vi "16TVTI-ReadITCStatus.vi"(0 "ITC IO Info":T1={"Com Port"=1, "ISOBUS Address"=1, "GPIB Address"=1, "Communication"=enum."ISOBUS"}) -> (2 "Control Channel":i16, 3 "System Status":i16, 4 "Auto heat":bool, 5 "ITC IO Info":T1={"Com Port"=1, "ISOBUS Address"=1, "GPIB Address"=1, "Communication"=enum."ISOBUS"}, 6 "Auto Needle Valve":bool, 8 "Sweeping":bool, 10 "Initialising Needle Valve":bool, 11 "Tuning?":bool, 13 "Auto PID":bool, 14 "Lock":bool, 15 "Remote":bool)   [LabVIEW 2019]
doc: "Reads the status of the ITC."
uses:
  Equipment/Oxford Software/Oxsoft/ITCSUBS.LLB/ITCIO.ctl
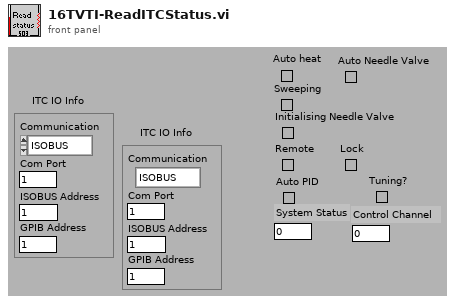
[diagram p1: front panel]
types:
  T1 = typedef "ITCIO.ctl" = cluster{"Com Port":i32, "ISOBUS Address":i32, "GPIB Address":i16, "Communication":enum16{"RS232", "ISOBUS", "GPIB", "Gateway"}}
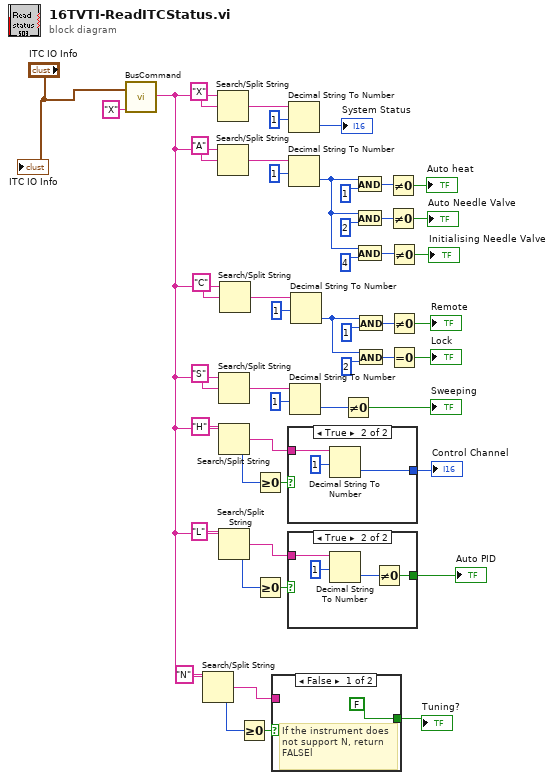
[diagram p0: block diagram]
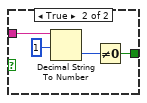
[diagram p2: hidden frame]
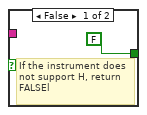
[diagram p3: hidden frame]
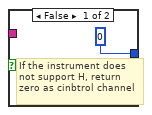
[diagram p4: hidden frame]
diagram:
  n1 = call "BusCommand.vi"("Command"="X", "Instrument address (in)"="ITC IO Info") -> ("Reply"=w7:string)  [unwired: 1 out]
  n2 = Search/Split String(string=w7, search string/char (-)="N") -> (match + rest of string=w6:string, offset of match=w4:i32)  [unwired: 1 in, 1 out]
  n3 = Search/Split String(string=w7, search string/char (-)="X") -> (match + rest of string=w48:string)  [unwired: 1 in, 2 out]
  n4 = Search/Split String(string=w7, search string/char (-)="A") -> (match + rest of string=w44:string)  [unwired: 1 in, 2 out]
  n5 = Search/Split String(string=w7, search string/char (-)="S") -> (match + rest of string=w26:string)  [unwired: 1 in, 2 out]
  n6 = Search/Split String(string=w7, search string/char (-)="H") -> (match + rest of string=w14:string, offset of match=w16:i32)  [unwired: 1 in, 1 out]
  n7 = Search/Split String(string=w7, search string/char (-)="L") -> (match + rest of string=w9:string, offset of match=w11:i32)  [unwired: 1 in, 1 out]
  n8 = Search/Split String(string=w7, search string/char (-)="C") -> (match + rest of string=w34:string)  [unwired: 1 in, 2 out]
  n9 = Greater Or Equal To 0?(x=w4) -> (x >= 0?=w5:bool)
  n10 = Greater Or Equal To 0?(x=w16) -> (x >= 0?=w15:bool)
  n11 = Greater Or Equal To 0?(x=w11) -> (x >= 0?=w10:bool)
  n12 = case shown="False" w5 {
    tunnel: w6 -> [_ w54]
    tunnel: [FALSE w52] -> w2
    frame False {
      # "If the instrument does\nnot support N, return\nFALSEl"
    }
    frame True {
      n13 = Decimal String To Number(string=w54, offset=1) -> (number=w53:i32)  [unwired: 1 in, 1 out]
      n14 = Not Equal To 0?(x=w53) -> (x != 0?=w52:bool)
    }
  }
  "Tuning?" <- w2
  n15 = case shown="True" w15 {
    tunnel: w14 -> [_ w58]
    tunnel: [0 w57] -> w13
    frame False {
      # "If the instrument does\nnot support H, return\nzero as cinbtrol channel"
    }
    frame True {
      n16 = Decimal String To Number(string=w58, offset=1) -> (number=w57:i32)  [unwired: 1 in, 1 out]
    }
  }
  "Control Channel" <- w13
  n17 = case shown="True" w10 {
    tunnel: w9 -> [_ w63]
    tunnel: [FALSE w61] -> w8
    frame False {
      # "If the instrument does\nnot support H, return\nFALSEl"
    }
    frame True {
      n18 = Decimal String To Number(string=w63, offset=1) -> (number=w62:i32)  [unwired: 1 in, 1 out]
      n19 = Not Equal To 0?(x=w62) -> (x != 0?=w61:bool)
    }
  }
  "Auto PID" <- w8
  n20 = Decimal String To Number(string=w48, offset=1) -> (number=→"System Status":i32)  [unwired: 1 in, 1 out]
  n21 = Decimal String To Number(string=w44, offset=1) -> (number=w37:i32)  [unwired: 1 in, 1 out]
  n22 = Decimal String To Number(string=w26, offset=1) -> (number=w24:i32)  [unwired: 1 in, 1 out]
  n23 = Decimal String To Number(string=w34, offset=1) -> (number=w30:i32)  [unwired: 1 in, 1 out]
  n24 = Not Equal To 0?(x=w24) -> (x != 0?=→"Sweeping":bool)
  n25 = And(x=w37, y=1) -> (x .and. y?=w42:i32)
  n26 = And(x=w37, y=2) -> (x .and. y?=w40:i32)
  n27 = And(x=w37, y=4) -> (x .and. y?=w38:i32)
  n28 = And(x=w30, y=1) -> (x .and. y?=w32:i32)
  n29 = And(x=w30, y=2) -> (x .and. y?=w31:i32)
  n30 = Not Equal To 0?(x=w42) -> (x != 0?=→"Auto heat":bool)
  n31 = Not Equal To 0?(x=w40) -> (x != 0?=→"Auto Needle Valve":bool)
  n32 = Not Equal To 0?(x=w38) -> (x != 0?=→"Initialising Needle Valve":bool)
  n33 = Not Equal To 0?(x=w32) -> (x != 0?=→"Remote":bool)
  n34 = Equal To 0?(x=w31) -> (x = 0?=→"Lock":bool)
  "ITC IO Info" <- "ITC IO Info"
